vi "Shift Tags for newly inserted tag.vi"(5 "Litt/BigEnd":bool, 6 "error in":errorcluster, 7 "Byte stream offset\nwhere new tag added":u32, 8 "Directories":T1[](array[typedef]), 9 "Image Data":u8[](array[numeric])) -> (0 "error out":errorcluster, 2 "Directories out":T1[](array[typedef]), 3 "Image Data Out":u8[](array[numeric]))   [LabVIEW 2015, in "Tiff reader.lvlib"]
doc: "This .vi shifts the tag Offsets for newly inserted tag that might be inserted before the tags. or their pointer locations."
uses:
  Tiff reader.lvlib
  FieldTypes.ctl
  IFD Entry.ctl
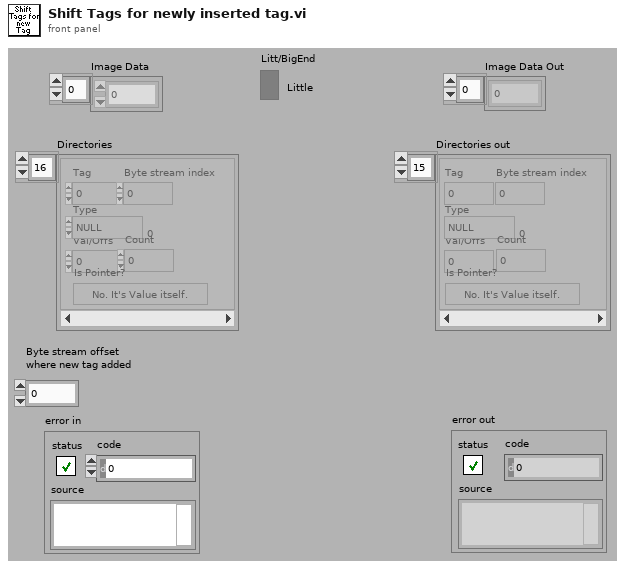
[diagram p1: front panel]
types:
  T1 = typedef "Tiff reader.lvlib/IFD Entry.ctl" = cluster{"Tag":u16, "Type":T2, "Count":u32, "Val/Offs":u32, "Is Pointer?":bool, "Byte stream index":i32}
  T2 = typedef "Tiff reader.lvlib/FieldTypes.ctl" = enum16{"NULL", "U8", "ASCII7", "U16", "U32", "RATIONAL", "SByte(I8)", "Undef(8Bit)", "I16", "I32", "SRat(4B:4B)", "SGL(4Byte)", "DBL(8Byte)"}
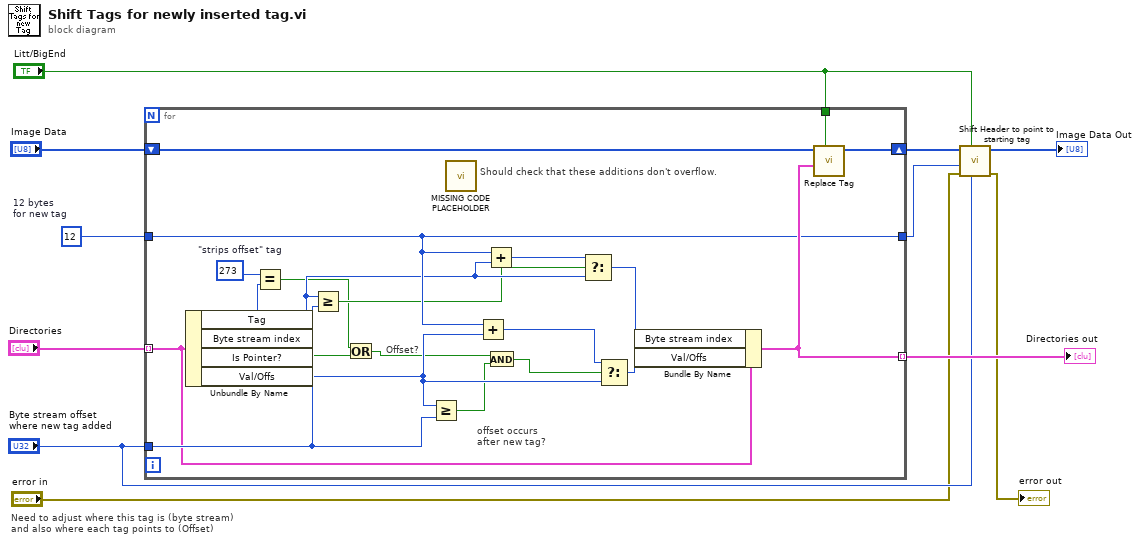
[diagram p0: block diagram]
diagram:
  w4 = 12  # 12 bytes  for new tag
  # "Need to adjust where this tag is (byte stream)\nand also where each tag points to (Offset)"
  n1 = for {
    tunnel: "Directories" -> [w31] mode=indexing
    tunnel: "Byte stream offset\nwhere new tag added" -> [w32]
    tunnel: [w27] -> w10 mode=indexing
    shift-right: [w28] -> w7
    shift-left: "Image Data" -> [w29]
    tunnel: "Litt/BigEnd" -> [w30]
    tunnel: [w26] -> w5
    tunnel: w4 -> [w26]
    w14 = u16 273  # "strips offset" tag
    # "Should check that these additions don't overflow."
    # "Offset?"
    # "offset occurs\nafter new tag?"
    n2 = Unbundle By Name(w31) -> ("Tag"=w13:u16, "Byte stream index"=w23:i32, "Is Pointer?"=w16:bool, "Val/Offs"=w18:u32)
    n3 = Equal?(x=w14, y=w13) -> (x = y?=w12:bool)
    n4 = Greater Or Equal?(x=w23, y=w32) -> (x >= y?=w21:bool)
    n5 = Or(x=w12, y=w16) -> (x .or. y?=w15:bool)
    n6 = Greater Or Equal?(x=w18, y=w32) -> (x >= y?=w17:bool)
    n7 = call "MISSING CODE PLACEHOLDER.vi"() -> ()  [unwired: 1 out]
    n8 = Add(x=w26, y=w18) -> (x+y=w20:u32)
    n9 = Add(x=w26, y=w23) -> (x+y=w25:i32)
    n10 = And(x=w15, y=w17) -> (x .and. y?=w19:bool)
    n11 = Select(t=w25, s=w21, f=w23) -> (s? t:f=w24:i32)
    n12 = Select(t=w20, s=w19, f=w18) -> (s? t:f=w22:u32)
    n13 = Bundle By Name(cluster=w31, "Byte stream index"=w24, "Val/Offs"=w22) -> (w27:T1)
    n14 = call "Replace Tag.vi"("Litt/BigEnd"=w30, "Tag"=w27, "Image Data in"=w29) -> ("Image Data Out"=w28:u8[])  [unwired: 2 in, 3 out]
  }
  "Directories out" <- w10
  n15 = call "Shift Header to point to starting tag.vi"("Byte stream offset\ninsertion point where \nnew data/tag added"="Byte stream offset\nwhere new tag added", "Litt/BigEnd"="Litt/BigEnd", "error in"="error in", "# bytes added\n(<0 means removed)"=w5, "Image Data"=w7) -> ("error out"=→"error out":errorcluster, "Image Data Out"=→"Image Data Out":u8[])  [unwired: 3 in, 2 out]
